vi "发送帧.vi"(10 "data":T1 {"数组"."标识" items=["N"=1, "T"=2, "L"=3, "D"=4, "Z"=5, "M"=6, "hd"=7]; "数组"."污染物" items=["水温"=1, "浊度"=2, "DO"=3, "pH"=4, "ORP"=5, "比电导率"=6, "叶绿素a"=7, "氨氮"=8, "亚硝氮"=9, "硫化物"=10, "电压"=11, "温度"=12, "湿度"=13, "GPS经度"=14, "GPS纬度"=15, "BD经度"=16, "BD纬度"=17]; "数据类别" items=["水样数据"=0, "标样数据"=1, "零点核查数据"=2, "跨度核查数据"=3, "环境变量"=4, "水样数据补传"=16, "标样核查数据补传"=17, "零点核查数据补传"=18, "跨度核查数据补传"=19]}, 11 "用户地址":string) -> (2 "报文长度":i32, 3 "字符串":string)   [LabVIEW 2016, in "环境动力监测库.lvlib" / "NMEA.lvlib"]
uses:
  NMEA.lvlib
panel:
  out "输出数组":u8[](array[numeric]) format="%02xH"
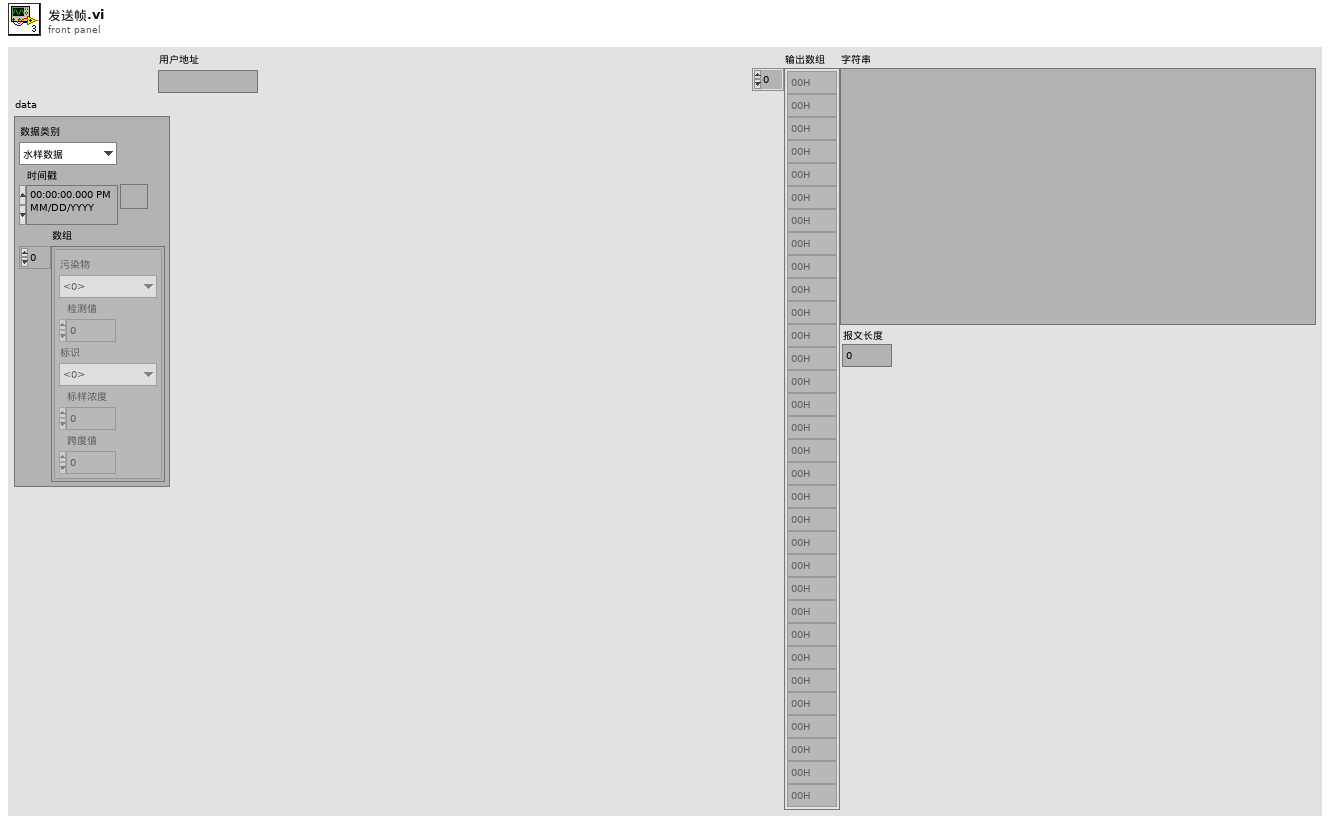
[diagram p1: front panel]
types:
  T1 = cluster{"数据类别":u16, "时间戳":timestamp, "数组":cluster{"污染物":u16, "检测值":dbl, "标识":u16, "标样浓度":dbl, "跨度值":dbl}[]}
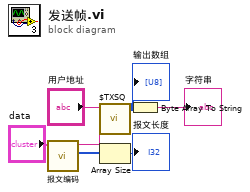
[diagram p0: block diagram]
diagram:
  n1 = call "报文编码.vi"("data"="data") -> ("数组"=w2:u8[], "字符串"=w7:string)  [unwired: 9 in]
  n2 = call "$TXSQ.vi"("电文内容"=w7, "用户地址"="用户地址") -> ("输出数组"=w5:u8[])  [unwired: 8 in, 1 out]
  "输出数组" <- w5
  n3 = Array Size(array=w2) -> (size(s)=→"报文长度":i32)
  n4 = Byte Array To String(unsigned byte array=w5) -> (string=→"字符串":string)
